vi "asap_micron_loop.vi"(4 "ASAP config":T1, 5 "error in":errorcluster, 8 "Micron config":T4) -> (0 "error out":errorcluster)   [LabVIEW 2014]
uses:
  initialization/micron_config.ctl
  manipulator/squiggle/Host/i2c_interface.ctl
  manipulator/squiggle/Host/fpga_reference.ctl
  testing/Micron params.ctl
  testing/stimulus.ctl
  testing/injection_point.ctl
  filtering/goal_loop_parms.ctl
  testing/mode_conrols.ctl
  testing/manipulator_cal.ctl
  asap/labview/testing/probe_calibration.ctl
  host/network_params.ctl
  sq_control_params.ctl
  decoupled_gain.ctl
  estimation_controls.ctl
  asap/labview/initialization/configuration.ctl
  asap/labview/initialization/asap_calibration.ctl
  <vilib>/Analysis/Matrix/Datatypes/RealMatrix.ctl
  <vilib>/Platform/TimedLoop/XDataNode/timing_clust.ctl
  <vilib>/Platform/TimedLoop/XDataNode/nitl_modes.ctl
  <vilib>/Platform/TimedLoop/XDataNode/wakeup.ctl
  initialization/micron_globals.vi
  <vilib>/Platform/TimedLoop/XDataNode/XDataNode.xnode
  <vilib>/NI_Real-Time Target Support.lvlib
  <vilib>/Platform/TimedLoop/XDataNode/XDNodeRunTimeDep.lvlib
  <vilib>/Analysis/Matrix/NI_Matrix.lvlib
panel:
  out "Each part":dbl[](array[numeric]) format="%#.1f"
  in  "Handle lights hold":bool
  in  "Light stimulus injection":i32
  in  "Times late":i32
  out "Cumulative":dbl[](array[numeric]) format="%#.1f"
  in  "Stop after profile":bool
  in  "Profile iterations":i32=30000
  out "total time histogram":T7(graph)
  out "cumulative times (uS)":dbl[][](graph)
  # "Times (us)"
  # "If \"Injection point\" is \"Light\", then we inject at ASAP light position, starting at the specified light."
  # "When true, freeze handle light position."
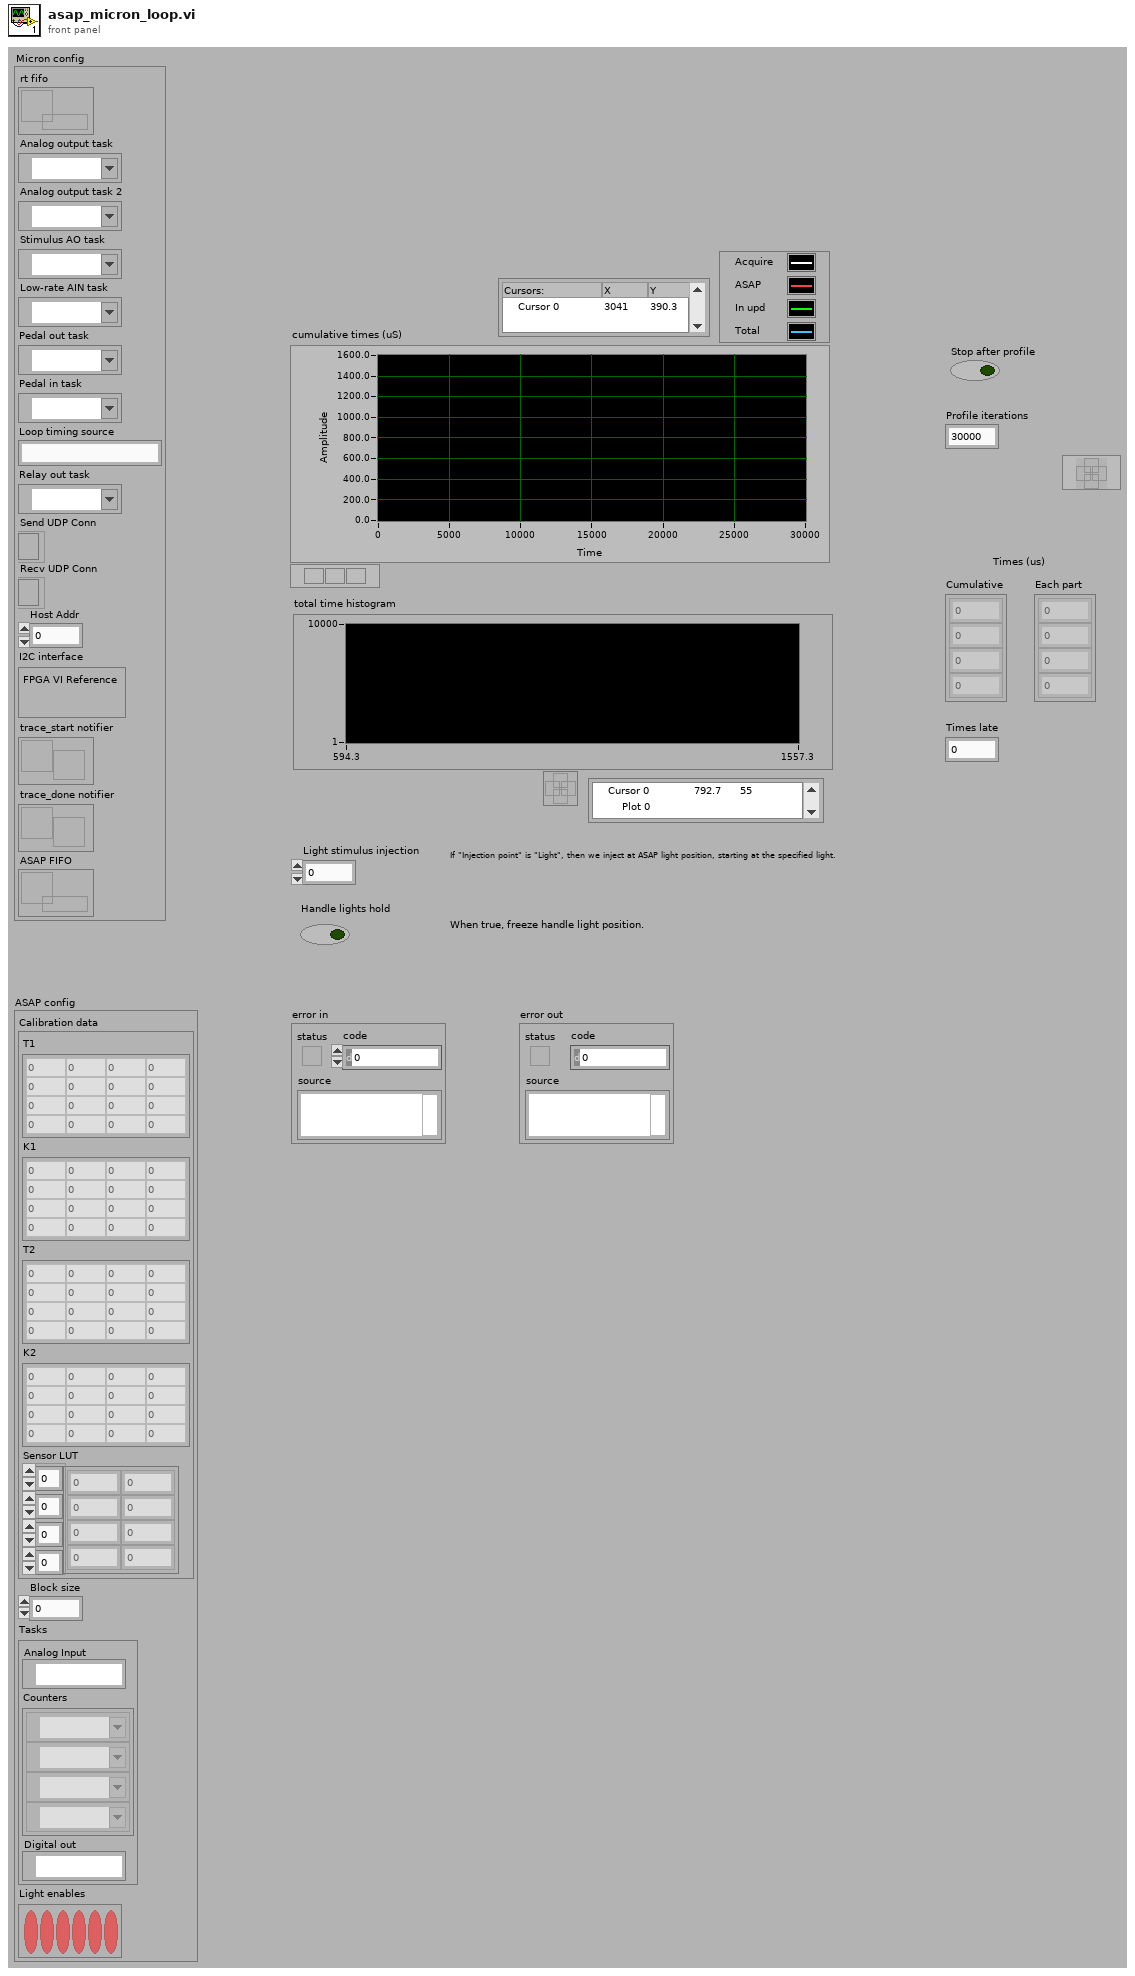
[diagram p1: front panel]
types:
  T1 = typedef "configuration.ctl" = cluster{"Calibration data":T2, "Block size":i32, "Tasks":cluster{"Analog Input":refnum<k21>, "Counters":refnum<k21>[], "Digital out":refnum<k21>}, "Light enables":bool[]}
  T2 = typedef "asap_calibration.ctl" = cluster{"T1":T3, "K1":T3, "T2":T3, "K2":T3, "Sensor LUT":sgl[][][][]}
  T3 = typedef "NI_Matrix.lvlib/RealMatrix.ctl" = dbl[][]
  T4 = typedef "micron_config.ctl" = cluster{"rt fifo":refnum<k33>, "Analog output task":refnum<k21>, "Analog output task 2":refnum<k21>, "Stimulus AO task":refnum<k21>, "Low-rate AIN task":refnum<k21>, "Pedal out task":refnum<k21>, "Pedal in task":refnum<k21>, "Loop timing source":string, "Relay out task":refnum<k21>, "Send UDP Conn":refnum<k16>, "Recv UDP Conn":refnum<k16>, "Host Addr":u32, "I2C interface":T5, "trace_start notifier":refnum<notifier>, "trace_done notifier":refnum<notifier>, "ASAP FIFO":refnum<k33>}
  T5 = typedef "i2c_interface.ctl" = cluster{"FPGA VI Reference":T6}
  T6 = typedef "fpga_reference.ctl" = refnum<k20>
  T7 = cluster{"X Values":dbl[], "Histogram: h(x)":i32[]}
  T8 = typedef "Micron params.ctl" = cluster{"Stimulus":T9, "Goal Filter A":T11, "Mode controls":T12, "Manipulator type":enum16{"Current piezo", "Voltage piezo"}, "Manipulator calibration":T13, "Network":T15, "Goal Filter B":T11, "Cancellation":T16, "Transition time":sgl, "Estimation":T18}
  T9 = typedef "stimulus.ctl" = cluster{"Type":enum16{"Off", "Step", "Sine", "Triangle", "Arbitrary"}, "Phase":dbl, "Amplitude":sgl[], "Injection point":T10, "Closed loop":bool, "Offset":sgl[], "Tip -> world":bool, "Frequency":dbl, "Length":dbl}
  T10 = typedef "injection_point.ctl" = enum16{"Total pose", "V limiter", "Goal ", "Link position", "KF link position", "Inverse kin", "Link goal", "Link error", "Controller", "Output", "Drive", "Light"}
  T11 = typedef "goal_loop_parms.ctl" = cluster{"Speedup max":sgl, "Speedup thresh":sgl, "Speedup nonlin":sgl, "Filters":cluster{"Lower Fc":sgl, "Lower Q":sgl, "Scale factor":sgl, "Upper Fc":sgl, "Upper Q":sgl, "V limit":sgl, "V limit range":sgl}[]}
  T12 = typedef "mode_conrols.ctl" = cluster{"Hold":bool, "Cancellation":bool, "Goal filter":bool, "Trigger":bool}
  T13 = typedef "manipulator_cal.ctl" = cluster{"Tool offsets":sgl[][], "Tip light calibration":T14, "Handle light calibration":T14, "Base pivots":sgl[][], "Output pivots":sgl[][], "Length center":sgl, "Workspace height":sgl[], "Workspace diameter":sgl[], "Linearization":sgl[][], "Stack travel":sgl, "Saturation pos":sgl, "Inverse filters":cluster{"filter structure":enum32{"IIR 2nd Order", "IIR 4th Order"}, "Reverse Coefficients":dbl[], "Forward Coefficients":dbl[]}[]}
  T14 = typedef "probe_calibration.ctl" = sgl[][]
  T15 = typedef "network_params.ctl" = cluster{"Remote Host":string, "Send Status":bool, "Send Port":u16, "Recv Commands":bool, "Recv Port":u16}
  T16 = typedef "sq_control_params.ctl" = cluster{"KP":T17, "KI":sgl, "KD":T17, "Max vel":sgl, "Max acc":sgl, "Int error limit":sgl, "RCM gain":sgl, "Bypass":bool, "Degraded gain":sgl}
  T17 = typedef "decoupled_gain.ctl" = cluster{"XY":sgl, "Rxy":sgl, "Z":sgl, "Rz":sgl}
  T18 = typedef "estimation_controls.ctl" = cluster{"Link":cluster{"Measure noise":dbl[], "Process noise":dbl[], "Alt process noise":dbl[], "Alt turnoff cycles":i32, "Innovation limit":dbl[], "Residue threshold":dbl, "Enable":bool}, "Handle":cluster{"Measure noise":dbl[], "Process noise":dbl[], "State limits":dbl[], "Innovation limit":dbl[], "Prediction Lookahead":sgl, "Enable":bool}}
  T19 = typedef "XDNodeRunTimeDep.lvlib/timing_clust.ctl" = cluster{"Expected End [f-1]":u64, "Actual End [f-1]":u64, "Finished Late? [f-1]":bool, "Expected End [i-1]":u64, "Actual End [i-1]":u64, "Finished Late? [i-1]":bool, "Expected Start [i]":u64, "Actual Start [i]":u64, "Expected Start [f]":u64, "Actual Start [f]":u64, "Source Name":string, "Structure Name":string, "Period":i64, "Deadline":i64, "Offset":i64, "Start":i64, "Priority":i32, "Timeout":i32, "Mode":T20, "Wakeup Reason":T21, "Error":errorcluster, "Source Type":string, "Secondary Source Type":string, "Global End Time":u64, "Global Start Time":u64, "Frame Duration":u64, "Iteration Duration":u64, "Assigned CPU":i32, "I/O Scan Engine Mode":u32}
  T20 = typedef "XDNodeRunTimeDep.lvlib/nitl_modes.ctl" = enum32{"No Change", "Process missed periods, maintain original phase", "Discard missed periods, maintain original phase", "Process missed periods, ignore original phase", "Discard missed periods, ignore original phase"}
  T21 = typedef "XDNodeRunTimeDep.lvlib/wakeup.ctl" = enum32{"Normal", "Aborted", "Asynchronous wakeup", "Timing source error", "Timed loop error", "Timeout"}
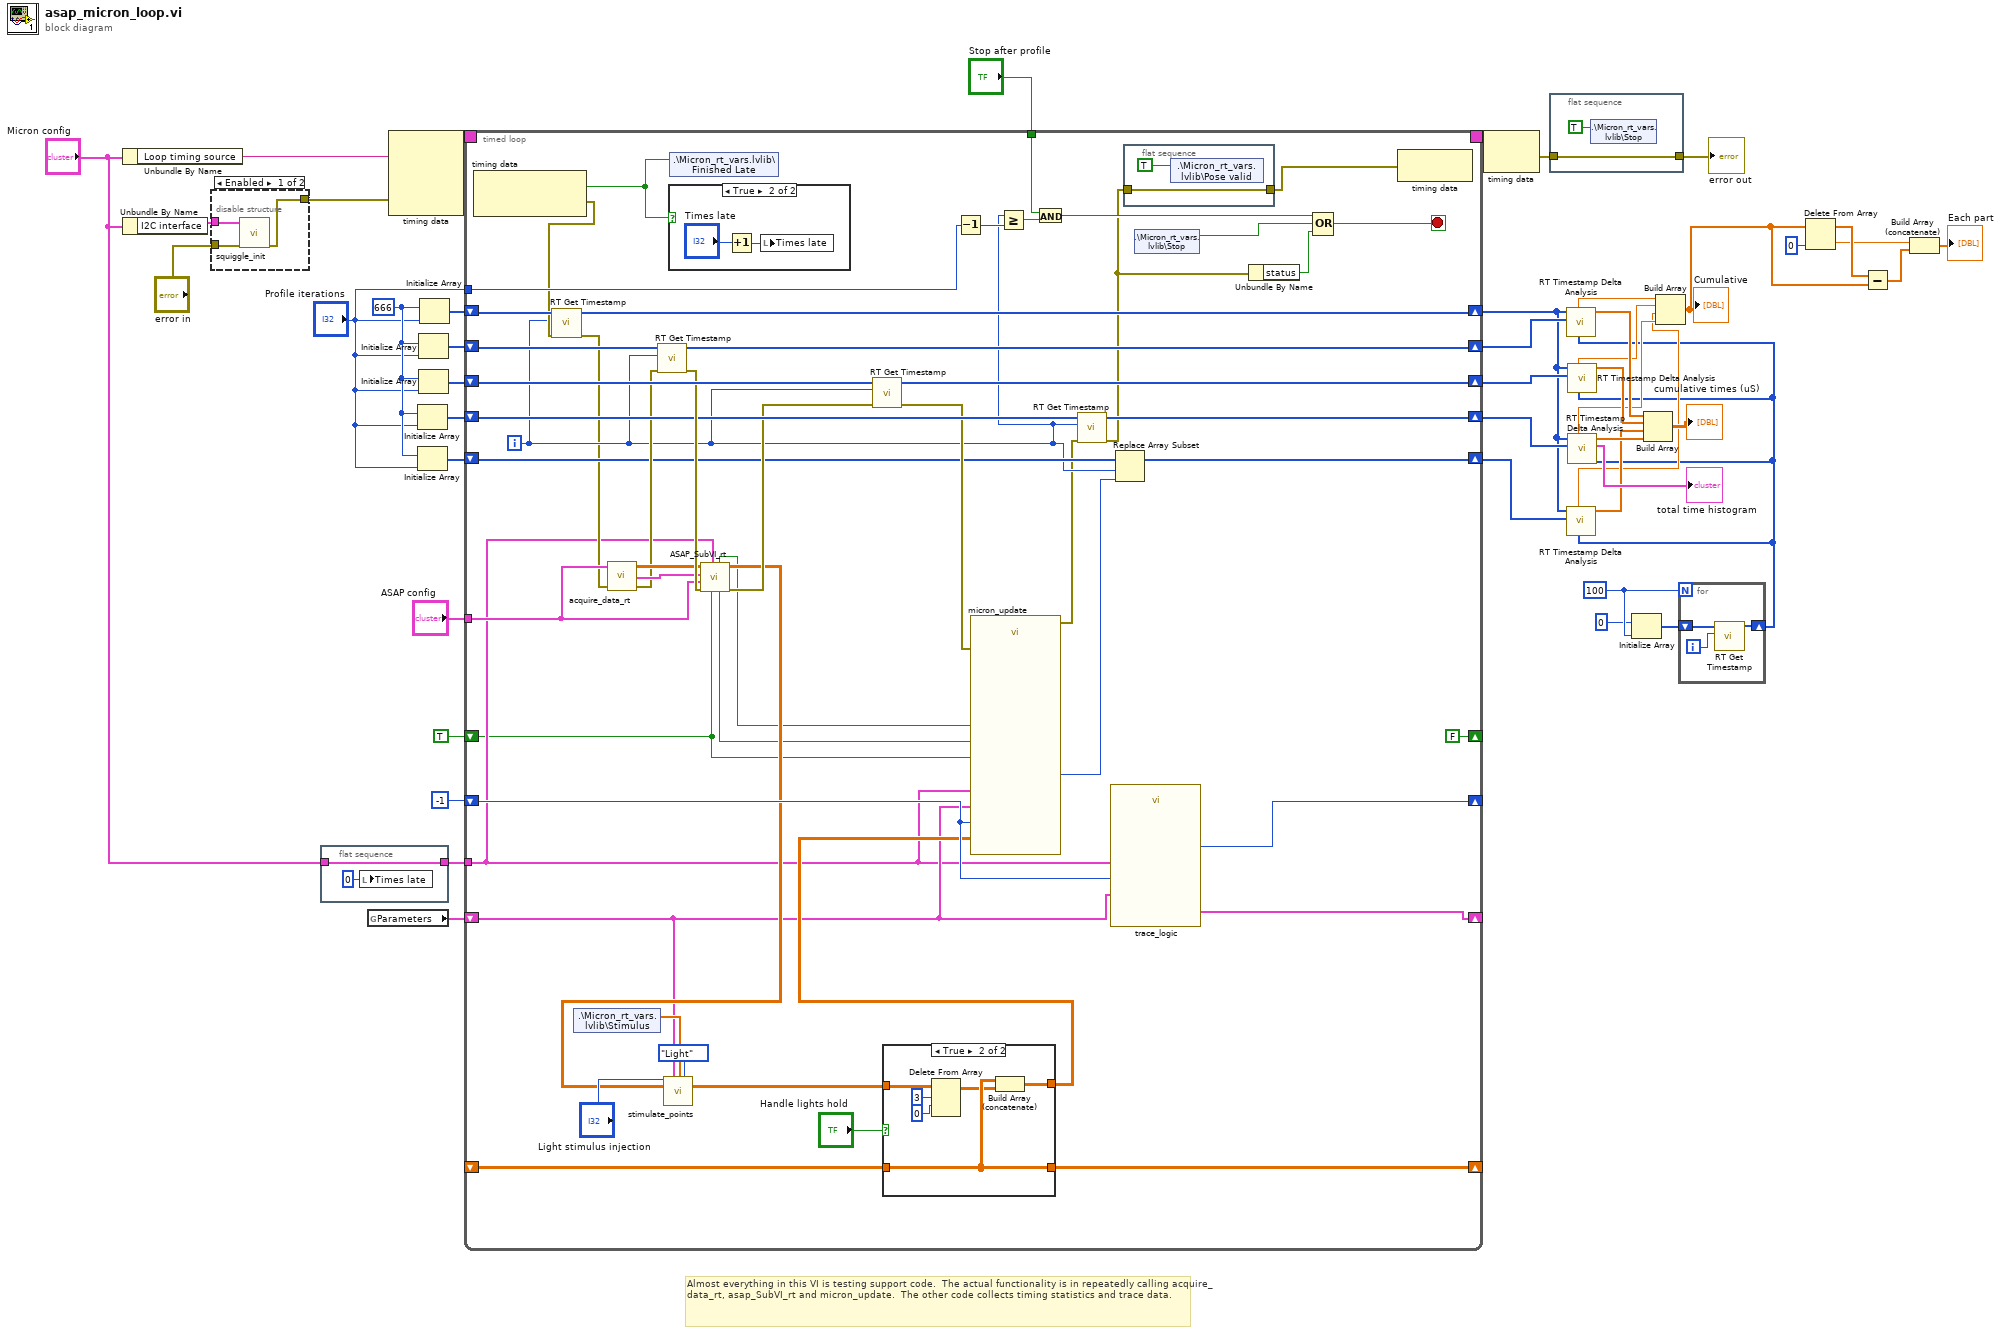
[diagram p0: block diagram]
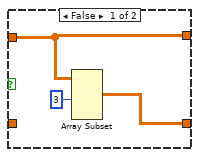
[diagram p3: hidden frame]
diagram:
  w29 = u64 666 ("element")
  w40 = 100
  # "Almost everything in this VI is testing support code.  The actual functionality is in repeatedly calling acquire_data_rt, asap_SubVI_rt and micron_update.  The other code collects timing statistics and trace data."
  n1 = Unbundle By Name("Micron config") -> ("Loop timing source"=w16:string)
  n2 = Unbundle By Name("Micron config") -> ("I2C interface"=w10:T5)
  n3 = disable-structure shown="Enabled" {
    disable-tunnel: w10 -> [w50 _]
    disable-tunnel: "error in" -> [w49 _]
    disable-tunnel: [w48 _] -> w8
    frame Enabled {
      n4 = call "squiggle_init.vi"("Error in"=w49, "I2C interface"=w50) -> ("Error out"=w48:errorcluster)  [unwired: 9 in]
    }
    frame Disabled {
    }
  }
  n5 = flat-sequence {
    tunnel: "Micron config" -> [w52]
    tunnel: [w52] -> w15
    frame #0 {
      n6 = local write "Times late"(0 ("Times late")) -> ()
    }
  }
  n7 = global read "micron_globals.vi" "Parameters"() -> (w11:T8)
  n8 = node-c288(w16, w8) -> (w18:T19)  [unwired: 2 out]
  n9 = Initialize Array(w29, "Profile iterations") -> (w37:u64[])
  n10 = Initialize Array(w29, "Profile iterations") -> (w27:u64[])
  n11 = Initialize Array(w29, "Profile iterations") -> (w45:u64[])
  n12 = Initialize Array(w29, "Profile iterations") -> (w46:u64[])
  n13 = Initialize Array(w29, "Profile iterations") -> (w47:u64[])
  n14 = timed-loop "deterministic loop" {
    tunnel: "ASAP config" -> [w91]
    tunnel: w15 -> [w56]
    shift-right: [w102] -> w36
    shift-left: w45 -> [w103]
    shift-right: [w100] -> w41
    shift-left: w46 -> [w101]
    tunnel: "Profile iterations" -> [w98]
    shift-right: [w95] -> w26
    shift-left: w47 -> [w96]
    tunnel: "Stop after profile" -> [w89]
    shift-right: [w87] -> w34
    shift-left: w37 -> [w88]
    shift-right: [w85] -> _
    shift-left: -1 ("trace index") -> [w77]
    shift-right: [FALSE ("Saturation")] -> _
    shift-left: TRUE ("Saturation") -> [w55]
    shift-right: [w75] -> w25
    shift-left: w27 -> [w76]
    shift-right: [w68] -> _
    shift-left: w11 -> [w58]
    timing: w18 -> [_]
    timing-out: [_] -> w17
    shift-right: [w60] -> _
    shift-left: _ -> [w62]
    i -> [w74]
    stop <- w94 stop-if-true
    n15 = node-c288() -> (w70:bool, w79:errorcluster)  [unwired: 1 out]
    n16 = call <vilib>:"RT Get Timestamp.vi"("error in (no error)"=w79, "iteration"=w74, "timestamp array in"=w96) -> ("error out"=w71:errorcluster, "timestamp array out"=w95:u64[])  [unwired: 7 out]
    n17 = shared-variable ".\\Micron_rt_vars.lvlib\\Stimulus"() -> (w65:sgl[])  [unwired: 2 out]
    n18 = call "acquire_data_rt.vi"("error in"=w71, "Configuration"=w91) -> ("error out"=w82:errorcluster, "timestamp"=w92:cluster{"t0":timestamp, "dt":dbl}, "Data"=w84:sgl[][])  [unwired: 1 out]
    n19 = call <vilib>:"RT Get Timestamp.vi"("error in (no error)"=w82, "iteration"=w74, "timestamp array in"=w103) -> ("error out"=w97:errorcluster, "timestamp array out"=w102:u64[])  [unwired: 7 out]
    n20 = case shown="True" w70 {
      frame False {
      }
      frame True {
        n21 = Increment(x="Times late") -> (x+1=w115:i32)
        n22 = local write "Times late"(w115) -> ()
      }
    }
    n23 = shared-variable ".\\Micron_rt_vars.lvlib\\Finished Late"(w70) -> ()  [unwired: 1 in, 1 out]
    n24 = call "ASAP_SubVI_rt.vi"("Reset"=w55, "Micron config"=w56, "error in"=w97, "Configuration"=w91, "Time in"=w92, "ADC data in"=w84) -> ("error out"=w86:errorcluster, "XYZ out"=w59:sgl[][], "Position valid"=w54:bool, "No pose"=w53:bool)  [unwired: 2 out]
    n25 = call "stimulate_points.vi"("Index"="Light stimulus injection", "Parameters"=w58, "Stimulus"=w65, "Injection point"=injection_point."Light", "Points in"=w59) -> ("Points out"=w64:sgl[][])  [unwired: 10 in]
    n26 = call <vilib>:"RT Get Timestamp.vi"("error in (no error)"=w86, "iteration"=w74, "timestamp array in"=w101) -> ("error out"=w83:errorcluster, "timestamp array out"=w100:u64[])  [unwired: 7 out]
    n27 = case shown="True" "Handle lights hold" {
      tunnel: w64 -> [w104 w112]
      tunnel: w62 -> [_ w109]
      tunnel: [w104 w107] -> w61
      tunnel: [w105 w109] -> w60
      frame False {
        n28 = Array Subset(array=w104, length (row)=3 ("length")) -> (w105:sgl[][])  [unwired: 3 in]
      }
      frame True {
        n29 = Delete From Array(array=w112, length=3, index (row)=0) -> (array with subset deleted=w108:sgl[][])  [unwired: 1 in, 1 out]
        n30 = Build Array (concatenate)(w109, w108) -> (w107:sgl[][])
      }
    }
    n31 = Decrement(x=w98) -> (x-1=w99:i32)
    n32 = call "micron_update.vi"("Position valid"=w54, "XYZ in"=w61, "Micron config"=w56, "error in"=w83, "No pose"=w53, "Reset"=w55, "Trace index"=w77, "Parameters"=w58) -> ("Timestamp"=w72:u64, "error out"=w73:errorcluster)  [unwired: 18 in]
    n33 = Greater Or Equal?(x=w74, y=w99) -> (x >= y?=w90:bool)
    n34 = And(x=w89, y=w90) -> (x .and. y?=w93:bool)
    n35 = call <vilib>:"RT Get Timestamp.vi"("error in (no error)"=w73, "iteration"=w74, "timestamp array in"=w88) -> ("error out"=w78:errorcluster, "timestamp array out"=w87:u64[])  [unwired: 7 out]
    n36 = call "trace_logic.vi"("Old trace index"=w77, "Parameters in"=w58, "Micron config"=w56) -> ("Parameters out"=w68:T8, "trace index"=w85:i32)  [unwired: 6 in]
    n37 = Replace Array Subset(array=w76, new element=w72, index=w74) -> (w75:u64[])
    n38 = flat-sequence {
      tunnel: w78 -> [w113]
      tunnel: [w113] -> w69
      frame #0 {
        n39 = shared-variable ".\\Micron_rt_vars.lvlib\\Pose valid"(TRUE ("Pose valid")) -> ()  [unwired: 2 out]
      }
    }
    n40 = shared-variable ".\\Micron_rt_vars.lvlib\\Stop"() -> (w80:bool)  [unwired: 2 out]
    n41 = Unbundle By Name(w78) -> ("status"=w81:bool)
    n42 = Compound Arithmetic op=OR(w93, w80, w81) -> (w94:bool)
    n43 = node-c288(w69) -> ()  [unwired: 1 out]
  }
  n44 = node-c288(w17) -> (w13:errorcluster)
  n45 = flat-sequence {
    tunnel: w13 -> [w123]
    tunnel: [w123] -> w12
    frame #0 {
      n46 = shared-variable ".\\Micron_rt_vars.lvlib\\Stop"(TRUE ("Stop")) -> ()  [unwired: 2 out]
    }
  }
  n47 = Initialize Array(u64 0 ("element"), w40) -> (w39:u64[])
  n48 = for {
    N: w40 -> [_]
    shift-right: [w125] -> w22
    shift-left: w39 -> [w127]
    i -> [w126]
    n49 = call <vilib>:"RT Get Timestamp.vi"("iteration"=w126, "timestamp array in"=w127) -> ("timestamp array out"=w125:u64[])  [unwired: 1 in, 8 out]
  }
  n50 = call "RT Timestamp Delta Analysis.vi"("calibration array"=w22, "timestamp array 2"=w36, "timestamp array 1"=w26) -> ("execution times (uS)"=w42:dbl[], "mean time (uS)"=w32:dbl)  [unwired: 3 in, 4 out]
  n51 = call "RT Timestamp Delta Analysis.vi"("calibration array"=w22, "timestamp array 2"=w25, "timestamp array 1"=w26) -> ("execution times (uS)"=w24:dbl[], "mean time (uS)"=w23:dbl)  [unwired: 3 in, 4 out]
  n52 = call "RT Timestamp Delta Analysis.vi"("calibration array"=w22, "timestamp array 2"=w41, "timestamp array 1"=w26) -> ("execution times (uS)"=w43:dbl[], "mean time (uS)"=w31:dbl)  [unwired: 3 in, 4 out]
  n53 = call "RT Timestamp Delta Analysis.vi"("calibration array"=w22, "timestamp array 2"=w34, "timestamp array 1"=w26) -> ("execution histogram"=→"total time histogram":T7, "execution times (uS)"=w33:dbl[], "mean time (uS)"=w30:dbl)  [unwired: 3 in, 3 out]
  n54 = Build Array(w42, w43, w24, w33) -> (→"cumulative times (uS)":dbl[][])
  n55 = Build Array(w32, w31, w23, w30) -> (w4:dbl[])
  "Cumulative" <- w4
  n56 = Delete From Array(array=w4, index=0) -> (deleted portion=w2:dbl, array with subset deleted=w5:dbl[])  [unwired: 1 in]
  n57 = Subtract(x=w5, y=w4) -> (x-y=w3:dbl[])
  n58 = Build Array (concatenate)(w2, w3) -> (→"Each part":dbl[])
  "error out" <- w12
